vi "Scan Rock Grid.vi"(1 "Rock Scan Trace":string) -> (0 "Rock Grid":set{cdb}(c389))   [LabVIEW 2020, in "AoC 2022.lvlib"]
uses:
  AoC 2022.lvlib
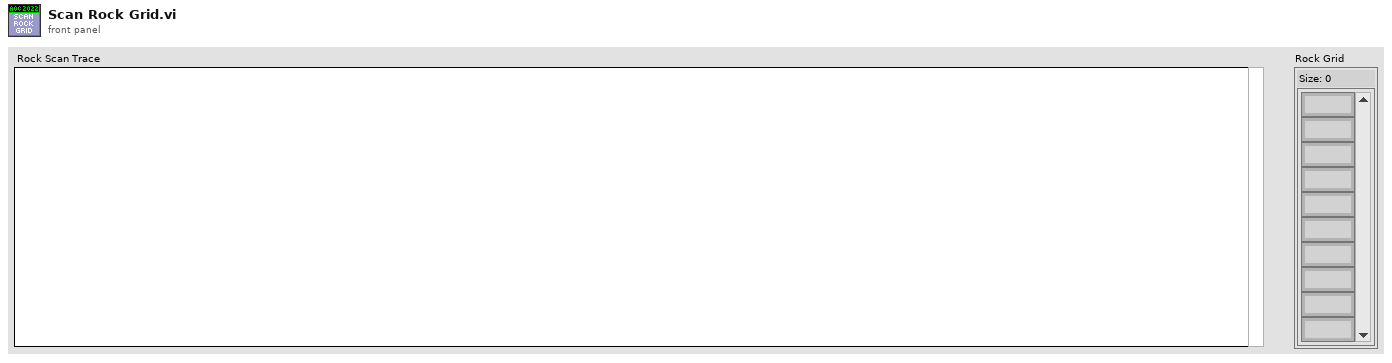
[diagram p1: front panel]
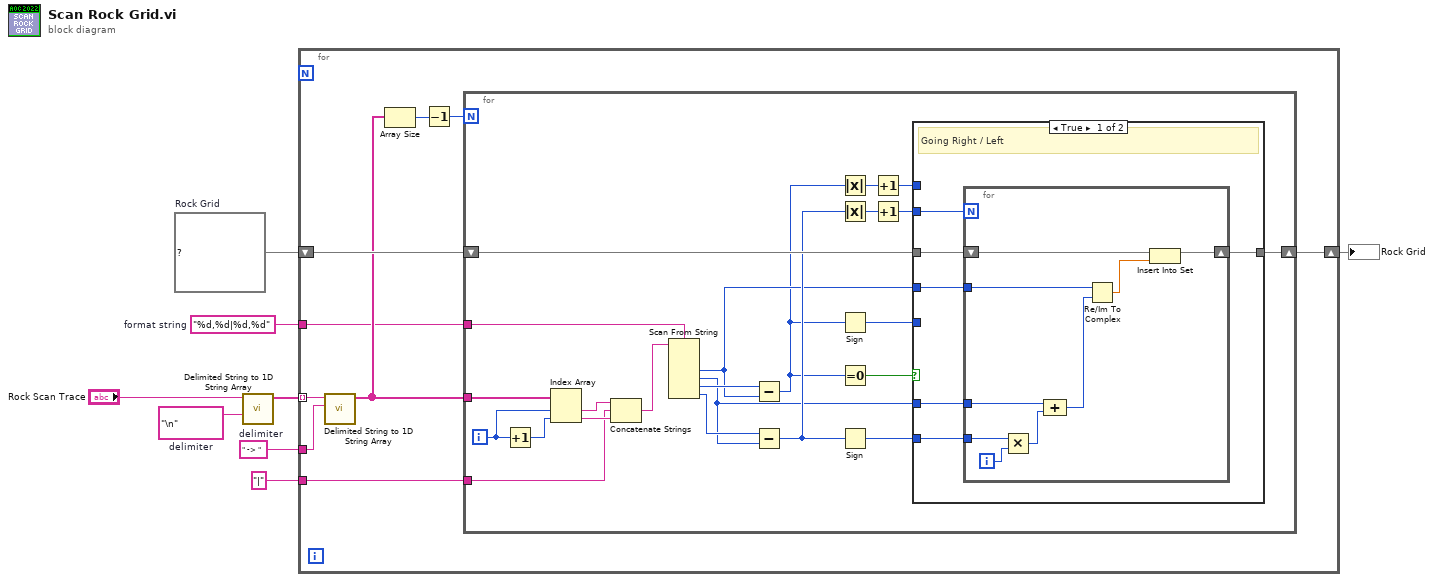
[diagram p0: block diagram]
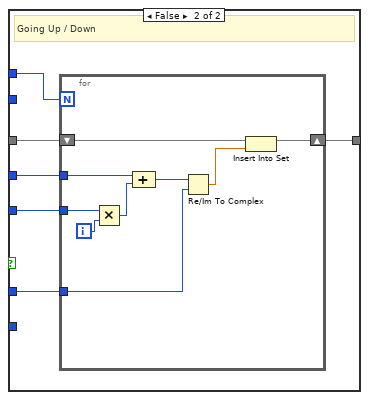
[diagram p2: hidden frame]
diagram:
  w6 = "%d,%d|%d,%d"  # format string
  w4 = " -> "  # delimiter
  w3 = set{cdb} {}  # Rock Grid
  w1 = "\n"  # delimiter
  n1 = call <vilib>:"Delimited String to 1D String Array.vi"("delimiter"=w1, "delimited string"="Rock Scan Trace") -> ("string array"=w2:string[])  [unwired: 9 in]
  n2 = for {
    tunnel: w2 -> [w14] mode=indexing
    shift-right: [w16] -> w8
    shift-left: w3 -> [w17]
    tunnel: w4 -> [w15]
    tunnel: w6 -> [w10]
    tunnel: "|" -> [w9]
    n3 = call <vilib>:"Delimited String to 1D String Array.vi"("delimiter"=w15, "delimited string"=w14) -> ("string array"=w13:string[])  [unwired: 9 in]
    n4 = Array Size(array=w13) -> (size(s)=w12:i32)
    n5 = Decrement(x=w12) -> (x-1=w11:i32)
    n6 = for {
      N: w11 -> [_]
      tunnel: w13 -> [w38]
      shift-right: [w39] -> w16
      shift-left: w17 -> [w40]
      tunnel: w10 -> [w35]
      tunnel: w9 -> [w32]
      i -> [w37]
      n7 = Increment(x=w37) -> (x+1=w36:i32)
      n8 = Index Array(array=w38, index #1=w37, index #2=w36) -> (element #1=w33:string, element #2=w34:string)
      n9 = Concatenate Strings(w33, w32, w34) -> (w31:string)
      n10 = Scan From String(format string=w35, input string=w31) -> (output 1=w27:i32, output 2=w26:i32, output 3=w30:i32, output 4=w29:i32)  [unwired: 6 in, 3 out]
      n11 = Subtract(x=w30, y=w27) -> (x-y=w21:i32)
      n12 = Subtract(x=w29, y=w26) -> (x-y=w28:i32)
      n13 = Absolute Value(x=w21) -> (abs(x)=w22:i32)
      n14 = Absolute Value(x=w28) -> (abs(x)=w24:i32)
      n15 = Sign(1:w21) -> (0:w25:i32)
      n16 = Equal To 0?(x=w21) -> (x = 0?=w20:bool)
      n17 = Sign(1:w28) -> (0:w23:i32)
      n18 = Increment(x=w22) -> (x+1=w19:i32)
      n19 = Increment(x=w24) -> (x+1=w18:i32)
      n20 = case shown="True" w20 {
        tunnel: w40 -> [w46 w61]
        tunnel: [w45 w60] -> w39
        tunnel: w27 -> [w44 w56]
        tunnel: w26 -> [w43 w57]
        tunnel: w25 -> [_ w58]
        tunnel: w18 -> [w42 _]
        tunnel: w23 -> [w41 _]
        tunnel: w19 -> [_ w59]
        frame True {
          # "Going Right / Left"
          n21 = for {
            N: w42 -> [_]
            shift-right: [w54] -> w45
            shift-left: w46 -> [w55]
            tunnel: w43 -> [w53]
            tunnel: w41 -> [w49]
            tunnel: w44 -> [w52]
            i -> [w48]
            n22 = Multiply(x=w49, y=w48) -> (x*y=w47:i32)
            n23 = Compound Arithmetic op=ADD(w53, w47) -> (w51:i32)
            n24 = Re/Im To Complex(1:w51, 2:w52) -> (0:w50:cdb)
            n25 = Insert Into Set(10:w50, 11:w55) -> (3:w54:set{cdb})  [unwired: 1 out]
          }
        }
        frame False {
          # "Going Up / Down"
          n26 = for {
            N: w59 -> [_]
            shift-right: [w69] -> w60
            shift-left: w61 -> [w70]
            tunnel: w56 -> [w68]
            tunnel: w58 -> [w62]
            tunnel: w57 -> [w65]
            i -> [w67]
            n27 = Multiply(x=w62, y=w67) -> (x*y=w63:i32)
            n28 = Compound Arithmetic op=ADD(w68, w63) -> (w64:i32)
            n29 = Re/Im To Complex(1:w65, 2:w64) -> (0:w66:cdb)
            n30 = Insert Into Set(10:w66, 11:w70) -> (3:w69:set{cdb})  [unwired: 1 out]
          }
        }
      }
    }
  }
  "Rock Grid" <- w8
